vi "VI Tree.vi"   [LabVIEW 2015, in "KEYENCE LJ-X8000A.lvlib"]
doc: "This is the instrument driver for the <INSTRUMENT NAME>. The VI Tree displays all the user-callable VIs of the instrument driver in an organized table."
uses:
  KEYENCE LJ-X8000A.lvlib
panel:
  # "(c) 2014 <Enter Company Name Here>.  ALL RIGHTS RESERVED."
  # "SEE DIAGRAM\nFOR VI TREE."
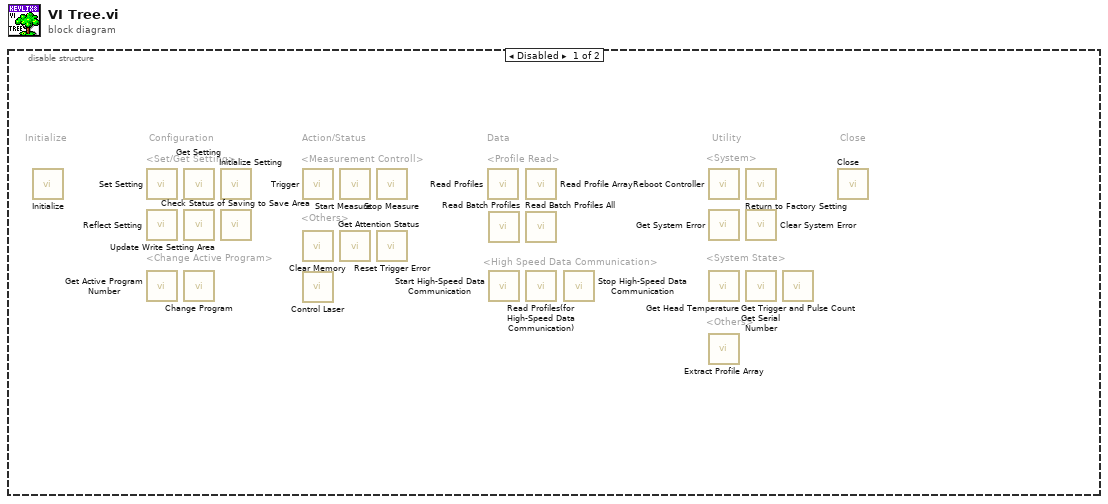
[diagram p0: block diagram]
diagram:
  n1 = disable-structure shown="Disabled" {
    frame Disabled {
      # "<Profile Read>"
      # "<High Speed Data Communication>"
      # "<Others>"
      # "<System State>"
      # "<System>"
      # "<Others>"
      # "<Measurement Controll>"
      # "<Change Active Program>"
      # "<Set/Get Setting>"
      # "Configuration"
      # "Utility"
      # "Data"
      # "Action/Status"
      # "Close"
      # "Initialize"
      n2 = call "Initialize.vi"() -> ()  [unwired: 10 in, 2 out]
      n3 = call "Set Setting.vi"() -> ()  [unwired: 9 in, 3 out]
      n4 = call "Reflect Setting.vi"() -> ()  [unwired: 9 in, 3 out]
      n5 = call "Get Active Program Number.vi"() -> ()  [unwired: 9 in, 3 out]
      n6 = call "Get Setting.vi"() -> ()  [unwired: 9 in, 3 out]
      n7 = call "Update Write Setting Area.vi"() -> ()  [unwired: 10 in, 2 out]
      n8 = call "Change Program.vi"() -> ()  [unwired: 10 in, 2 out]
      n9 = call "Initialize Setting.vi"() -> ()  [unwired: 10 in, 2 out]
      n10 = call "Check Status of Saving to Save Area.vi"() -> ()  [unwired: 9 in, 3 out]
      n11 = call "Trigger.vi"() -> ()  [unwired: 10 in, 2 out]
      n12 = call "Clear Memory.vi"() -> ()  [unwired: 10 in, 2 out]
      n13 = call "Control Laser.vi"() -> ()  [unwired: 10 in, 2 out]
      n14 = call "Start Measure.vi"() -> ()  [unwired: 10 in, 2 out]
      n15 = call "Get Attention Status.vi"() -> ()  [unwired: 11 in, 5 out]
      n16 = call "Stop Measure.vi"() -> ()  [unwired: 10 in, 2 out]
      n17 = call "Reset Trigger Error.vi"() -> ()  [unwired: 10 in, 2 out]
      n18 = call "Read Profiles.vi"() -> ()  [unwired: 7 in, 5 out]
      n19 = call "Read Batch Profiles.vi"() -> ()  [unwired: 7 in, 5 out]
      n20 = call "Start High-Speed Data Communication.vi"() -> ()  [unwired: 14 in, 2 out]
      n21 = call "Read Profile Array.vi"() -> ()  [unwired: 9 in, 7 out]
      n22 = call "Read Batch Profiles All.vi"() -> ()  [unwired: 8 in, 8 out]
      n23 = call "Read Profiles(for High-Speed Data Communication).vi"() -> ()  [unwired: 9 in, 7 out]
      n24 = call "Stop High-Speed Data Communication.vi"() -> ()  [unwired: 10 in, 2 out]
      n25 = call "Reboot Controller.vi"() -> ()  [unwired: 10 in, 2 out]
      n26 = call "Get System Error.vi"() -> ()  [unwired: 8 in, 4 out]
      n27 = call "Get Head Temperature.vi"() -> ()  [unwired: 11 in, 5 out]
      n28 = call "Extract Profile Array.vi"() -> ()  [unwired: 8 in, 4 out]
      n29 = call "Return to Factory Setting.vi"() -> ()  [unwired: 10 in, 2 out]
      n30 = call "Clear System Error.vi"() -> ()  [unwired: 10 in, 2 out]
      n31 = call "Get Serial Number.vi"() -> ()  [unwired: 8 in, 4 out]
      n32 = call "Get Trigger and Pulse Count.vi"() -> ()  [unwired: 8 in, 4 out]
      n33 = call "Close.vi"() -> ()  [unwired: 10 in, 2 out]
    }
    frame Enabled {
    }
  }
